vi "TSLIN_LIN_Schedule_Tab.vi"(8 "错误输入（无错误）":errorcluster, 10 "Data":T1={"Communication message"={"Sender"="", "receiver"="", "message"="", "data"=variant}, "LIN_Data"={"DLL_PATH"=path "", "Channels used"=1, "Funtiontype"=0, "Rx/TX"=enum."Rx", "Read message type"=enum."Receive&send messages", "async&sync"=enum."async", "sync_sendTimeout"=0, "LIN_SendHead"={"ALINIdxchn"=0, "ALINId"=0, "ALINDLC"=0}, "LIN_Set"={"Hardware Type"=3, "Hardware Subtype"=enum."TC1026", "AHwChannel"=0, "AAppChannel"=0, "ABaudrateKbps"=19.2, "AProtocol"=2, "AldHW"=0}, "LIN_DATA"={"Data0"=0, "Data1"=0, "Data2"=0, "Data3"=0, "Data4"=0, "Data5"=0, "Data6"=0, "Data7"=0}, "LIN_Set_Array"=[], "LDF"={"LDF Path"=path "", "LDF loading channel"=0}, "Blf_Log"={"Blf_Log_PATH"=path ""}, "LIN Scheduling Table Array"=[], "REC_Channel"=0}, "LIN Data array"=[], "error in"={"status"=FALSE, "code"=0, "source"=""}, "REC_Channel"=0, "AsynCall?"=FALSE, "DataBase_array"=refnum} {"REC_Channel" items=["CHN1", "CHN2", "CHN3", "CHN4", "CHN5", "CHN6", "CHN7", "CHN8", "CHN9", "CHN10", "CHN11", "CHN12", "CHN13", "CHN14", "CHN15", "CHN16", "CHN17", "CHN18", "CHN19", "CHN20", "CHN21", "CHN22", "CHN23", "CHN24", "CHN25", "CHN26", "CHN27", "CHN28", "CHN29", "CHN30", "CHN31", "CHN32"]; "LIN_Data"."REC_Channel" items=["CHN1", "CHN2", "CHN3", "CHN4", "CHN5", "CHN6", "CHN7", "CHN8", "CHN9", "CHN10", "CHN11", "CHN12", "CHN13", "CHN14", "CHN15", "CHN16", "CHN17", "CHN18", "CHN19", "CHN20", "CHN21", "CHN22", "CHN23", "CHN24", "CHN25", "CHN26", "CHN27", "CHN28", "CHN29", "CHN30", "CHN31", "CHN32"]; "LIN_Data"."LIN Scheduling Table Array"."LIN_Transmit"."Channel" items=["CHN1", "CHN2", "CHN3", "CHN4", "CHN5", "CHN6", "CHN7", "CHN8", "CHN9", "CHN10", "CHN11", "CHN12", "CHN13", "CHN14", "CHN15", "CHN16", "CHN17", "CHN18", "CHN19", "CHN20", "CHN21", "CHN22", "CHN23", "CHN24", "CHN25", "CHN26", "CHN27", "CHN28", "CHN29", "CHN30", "CHN31", "CHN32"]; "LIN_Data"."LIN Scheduling Table Array"."LIN_Transmit"."ID" format="%.0x"; "LIN_Data"."LIN Scheduling Table Array"."LIN_Transmit"."DLC" format="%.0x"; "LIN_Data"."LIN Scheduling Table Array"."LIN_Transmit"."Set_node_funtiontype" items=["MasterNode", "SlaveNode", "MonitorNote"]; "LIN_Data"."LDF"."LDF loading channel" items=["CHN1", "CHN2", "CHN3", "CHN4", "CHN5", "CHN6", "CHN7", "CHN8", "CHN9", "CHN10", "CHN11", "CHN12", "CHN13", "CHN14", "CHN15", "CHN16", "CHN17", "CHN18", "CHN19", "CHN20", "CHN21", "CHN22", "CHN23", "CHN24", "CHN25", "CHN26", "CHN27", "CHN28", "CHN29", "CHN30", "CHN31", "CHN32"]; "LIN_Data"."LIN_Set_Array"."Set_node_funtiontype" items=["MasterNode", "SlaveNode", "MonitorNote"]; "LIN_Data"."LIN_Set_Array"."Set"."Hardware Type" items=["BUS_UNKNOWN_TYPE", "TS_TCP_DEVICE", "XL_USB_DEVICE", "TS_USB_DEVICE", "PEAK_USB_DEVICE", "KVASER_USB_DEVICE", "ZLG_USB_DEVICE", "ICS_USB_DEVICE", "TS_TC1005_DEVICE", "CANABLE_USB_DEVICE", "TS_WIRELESS_OBD", "TS_USB_DEVICE_EX", "IXXAT_USB_DEVICE", "TS_ETH_IF_DEVICE", "TS_USB_IF_DEVICE", "BUS_DEV_TYPE_COUNT"]; "LIN_Data"."LIN_Set_Array"."Set"."AHwChannel" items=["CHN1", "CHN2", "CHN3", "CHN4", "CHN5", "CHN6", "CHN7", "CHN8", "CHN9", "CHN10", "CHN11", "CHN12", "CHN13", "CHN14", "CHN15", "CHN16", "CHN17", "CHN18", "CHN19", "CHN20", "CHN21", "CHN22", "CHN23", "CHN24", "CHN25", "CHN26", "CHN27", "CHN28", "CHN29", "CHN30", "CHN31", "CHN32"]; "LIN_Data"."LIN_Set_Array"."Set"."AAppChannel" items=["CHN1", "CHN2", "CHN3", "CHN4", "CHN5", "CHN6", "CHN7", "CHN8", "CHN9", "CHN10", "CHN11", "CHN12", "CHN13", "CHN14", "CHN15", "CHN16", "CHN17", "CHN18", "CHN19", "CHN20", "CHN21", "CHN22", "CHN23", "CHN24", "CHN25", "CHN26", "CHN27", "CHN28", "CHN29", "CHN30", "CHN31", "CHN32"]; "LIN_Data"."LIN_Set_Array"."Set"."AProtocol" items=["Lin_Protocol_13", "Lin_Protocol_20", "Lin_Protocol_21", "Lin_Protocol_J2602"]; "LIN_Data"."Funtiontype" items=["MasterNode", "SlaveNode", "MonitorNote"]; "LIN_Data"."LIN_SendHead"."ALINDLC" format="%.0x"; "LIN_Data"."LIN_SendHead"."ALINId" format="%.0x"; "LIN_Data"."LIN_SendHead"."ALINIdxchn" items=["CHN1", "CHN2", "CHN3", "CHN4", "CHN5", "CHN6", "CHN7", "CHN8", "CHN9", "CHN10", "CHN11", "CHN12", "CHN13", "CHN14", "CHN15", "CHN16", "CHN17", "CHN18", "CHN19", "CHN20", "CHN21", "CHN22", "CHN23", "CHN24", "CHN25", "CHN26", "CHN27", "CHN28", "CHN29", "CHN30", "CHN31", "CHN32"]; "LIN_Data"."LIN_Set"."Hardware Type" items=["BUS_UNKNOWN_TYPE", "TS_TCP_DEVICE", "XL_USB_DEVICE", "TS_USB_DEVICE", "PEAK_USB_DEVICE", "KVASER_USB_DEVICE", "ZLG_USB_DEVICE", "ICS_USB_DEVICE", "TS_TC1005_DEVICE", "CANABLE_USB_DEVICE", "TS_WIRELESS_OBD", "TS_USB_DEVICE_EX", "IXXAT_USB_DEVICE", "TS_ETH_IF_DEVICE", "TS_USB_IF_DEVICE", "BUS_DEV_TYPE_COUNT"]; "LIN_Data"."LIN_Set"."AHwChannel" items=["CHN1", "CHN2", "CHN3", "CHN4", "CHN5", "CHN6", "CHN7", "CHN8", "CHN9", "CHN10", "CHN11", "CHN12", "CHN13", "CHN14", "CHN15", "CHN16", "CHN17", "CHN18", "CHN19", "CHN20", "CHN21", "CHN22", "CHN23", "CHN24", "CHN25", "CHN26", "CHN27", "CHN28", "CHN29", "CHN30", "CHN31", "CHN32"]; "LIN_Data"."LIN_Set"."AAppChannel" items=["CHN1", "CHN2", "CHN3", "CHN4", "CHN5", "CHN6", "CHN7", "CHN8", "CHN9", "CHN10", "CHN11", "CHN12", "CHN13", "CHN14", "CHN15", "CHN16", "CHN17", "CHN18", "CHN19", "CHN20", "CHN21", "CHN22", "CHN23", "CHN24", "CHN25", "CHN26", "CHN27", "CHN28", "CHN29", "CHN30", "CHN31", "CHN32"]; "LIN_Data"."LIN_Set"."AProtocol" items=["Lin_Protocol_13", "Lin_Protocol_20", "Lin_Protocol_21", "Lin_Protocol_J2602"]; "LIN_Data"."Channels used" items=["1 Channel"=1, "2 Channels"=2, "3 Channels"=3, "4 Channels"=4, "5 Channels"=5]}, 11 "Sender":string="Demo") -> (0 "错误输出":errorcluster, 3 "Data out":T1={"Communication message"={"Sender"="", "receiver"="", "message"="", "data"=variant}, "LIN_Data"={"DLL_PATH"=path "", "Channels used"=1, "Funtiontype"=0, "Rx/TX"=enum."Rx", "Read message type"=enum."Receive&send messages", "async&sync"=enum."async", "sync_sendTimeout"=0, "LIN_SendHead"={"ALINIdxchn"=0, "ALINId"=0, "ALINDLC"=0}, "LIN_Set"={"Hardware Type"=3, "Hardware Subtype"=enum."TC1026", "AHwChannel"=0, "AAppChannel"=0, "ABaudrateKbps"=19.2, "AProtocol"=2, "AldHW"=0}, "LIN_DATA"={"Data0"=0, "Data1"=0, "Data2"=0, "Data3"=0, "Data4"=0, "Data5"=0, "Data6"=0, "Data7"=0}, "LIN_Set_Array"=[], "LDF"={"LDF Path"=path "", "LDF loading channel"=0}, "Blf_Log"={"Blf_Log_PATH"=path ""}, "LIN Scheduling Table Array"=[], "REC_Channel"=0}, "LIN Data array"=[], "error in"={"status"=FALSE, "code"=0, "source"=""}, "REC_Channel"=0, "AsynCall?"=FALSE, "DataBase_array"=refnum} {"REC_Channel" items=["CHN1", "CHN2", "CHN3", "CHN4", "CHN5", "CHN6", "CHN7", "CHN8", "CHN9", "CHN10", "CHN11", "CHN12", "CHN13", "CHN14", "CHN15", "CHN16", "CHN17", "CHN18", "CHN19", "CHN20", "CHN21", "CHN22", "CHN23", "CHN24", "CHN25", "CHN26", "CHN27", "CHN28", "CHN29", "CHN30", "CHN31", "CHN32"]; "LIN_Data"."REC_Channel" items=["CHN1", "CHN2", "CHN3", "CHN4", "CHN5", "CHN6", "CHN7", "CHN8", "CHN9", "CHN10", "CHN11", "CHN12", "CHN13", "CHN14", "CHN15", "CHN16", "CHN17", "CHN18", "CHN19", "CHN20", "CHN21", "CHN22", "CHN23", "CHN24", "CHN25", "CHN26", "CHN27", "CHN28", "CHN29", "CHN30", "CHN31", "CHN32"]; "LIN_Data"."LIN Scheduling Table Array"."LIN_Transmit"."Channel" items=["CHN1", "CHN2", "CHN3", "CHN4", "CHN5", "CHN6", "CHN7", "CHN8", "CHN9", "CHN10", "CHN11", "CHN12", "CHN13", "CHN14", "CHN15", "CHN16", "CHN17", "CHN18", "CHN19", "CHN20", "CHN21", "CHN22", "CHN23", "CHN24", "CHN25", "CHN26", "CHN27", "CHN28", "CHN29", "CHN30", "CHN31", "CHN32"]; "LIN_Data"."LIN Scheduling Table Array"."LIN_Transmit"."ID" format="%.0x"; "LIN_Data"."LIN Scheduling Table Array"."LIN_Transmit"."DLC" format="%.0x"; "LIN_Data"."LIN Scheduling Table Array"."LIN_Transmit"."Set_node_funtiontype" items=["MasterNode", "SlaveNode", "MonitorNote"]; "LIN_Data"."LDF"."LDF loading channel" items=["CHN1", "CHN2", "CHN3", "CHN4", "CHN5", "CHN6", "CHN7", "CHN8", "CHN9", "CHN10", "CHN11", "CHN12", "CHN13", "CHN14", "CHN15", "CHN16", "CHN17", "CHN18", "CHN19", "CHN20", "CHN21", "CHN22", "CHN23", "CHN24", "CHN25", "CHN26", "CHN27", "CHN28", "CHN29", "CHN30", "CHN31", "CHN32"]; "LIN_Data"."LIN_Set_Array"."Set_node_funtiontype" items=["MasterNode", "SlaveNode", "MonitorNote"]; "LIN_Data"."LIN_Set_Array"."Set"."Hardware Type" items=["BUS_UNKNOWN_TYPE", "TS_TCP_DEVICE", "XL_USB_DEVICE", "TS_USB_DEVICE", "PEAK_USB_DEVICE", "KVASER_USB_DEVICE", "ZLG_USB_DEVICE", "ICS_USB_DEVICE", "TS_TC1005_DEVICE", "CANABLE_USB_DEVICE", "TS_WIRELESS_OBD", "TS_USB_DEVICE_EX", "IXXAT_USB_DEVICE", "TS_ETH_IF_DEVICE", "TS_USB_IF_DEVICE", "BUS_DEV_TYPE_COUNT"]; "LIN_Data"."LIN_Set_Array"."Set"."AHwChannel" items=["CHN1", "CHN2", "CHN3", "CHN4", "CHN5", "CHN6", "CHN7", "CHN8", "CHN9", "CHN10", "CHN11", "CHN12", "CHN13", "CHN14", "CHN15", "CHN16", "CHN17", "CHN18", "CHN19", "CHN20", "CHN21", "CHN22", "CHN23", "CHN24", "CHN25", "CHN26", "CHN27", "CHN28", "CHN29", "CHN30", "CHN31", "CHN32"]; "LIN_Data"."LIN_Set_Array"."Set"."AAppChannel" items=["CHN1", "CHN2", "CHN3", "CHN4", "CHN5", "CHN6", "CHN7", "CHN8", "CHN9", "CHN10", "CHN11", "CHN12", "CHN13", "CHN14", "CHN15", "CHN16", "CHN17", "CHN18", "CHN19", "CHN20", "CHN21", "CHN22", "CHN23", "CHN24", "CHN25", "CHN26", "CHN27", "CHN28", "CHN29", "CHN30", "CHN31", "CHN32"]; "LIN_Data"."LIN_Set_Array"."Set"."AProtocol" items=["Lin_Protocol_13", "Lin_Protocol_20", "Lin_Protocol_21", "Lin_Protocol_J2602"]; "LIN_Data"."Funtiontype" items=["MasterNode", "SlaveNode", "MonitorNote"]; "LIN_Data"."LIN_SendHead"."ALINDLC" format="%.0x"; "LIN_Data"."LIN_SendHead"."ALINId" format="%.0x"; "LIN_Data"."LIN_SendHead"."ALINIdxchn" items=["CHN1", "CHN2", "CHN3", "CHN4", "CHN5", "CHN6", "CHN7", "CHN8", "CHN9", "CHN10", "CHN11", "CHN12", "CHN13", "CHN14", "CHN15", "CHN16", "CHN17", "CHN18", "CHN19", "CHN20", "CHN21", "CHN22", "CHN23", "CHN24", "CHN25", "CHN26", "CHN27", "CHN28", "CHN29", "CHN30", "CHN31", "CHN32"]; "LIN_Data"."LIN_Set"."Hardware Type" items=["BUS_UNKNOWN_TYPE", "TS_TCP_DEVICE", "XL_USB_DEVICE", "TS_USB_DEVICE", "PEAK_USB_DEVICE", "KVASER_USB_DEVICE", "ZLG_USB_DEVICE", "ICS_USB_DEVICE", "TS_TC1005_DEVICE", "CANABLE_USB_DEVICE", "TS_WIRELESS_OBD", "TS_USB_DEVICE_EX", "IXXAT_USB_DEVICE", "TS_ETH_IF_DEVICE", "TS_USB_IF_DEVICE", "BUS_DEV_TYPE_COUNT"]; "LIN_Data"."LIN_Set"."AHwChannel" items=["CHN1", "CHN2", "CHN3", "CHN4", "CHN5", "CHN6", "CHN7", "CHN8", "CHN9", "CHN10", "CHN11", "CHN12", "CHN13", "CHN14", "CHN15", "CHN16", "CHN17", "CHN18", "CHN19", "CHN20", "CHN21", "CHN22", "CHN23", "CHN24", "CHN25", "CHN26", "CHN27", "CHN28", "CHN29", "CHN30", "CHN31", "CHN32"]; "LIN_Data"."LIN_Set"."AAppChannel" items=["CHN1", "CHN2", "CHN3", "CHN4", "CHN5", "CHN6", "CHN7", "CHN8", "CHN9", "CHN10", "CHN11", "CHN12", "CHN13", "CHN14", "CHN15", "CHN16", "CHN17", "CHN18", "CHN19", "CHN20", "CHN21", "CHN22", "CHN23", "CHN24", "CHN25", "CHN26", "CHN27", "CHN28", "CHN29", "CHN30", "CHN31", "CHN32"]; "LIN_Data"."LIN_Set"."AProtocol" items=["Lin_Protocol_13", "Lin_Protocol_20", "Lin_Protocol_21", "Lin_Protocol_J2602"]; "LIN_Data"."Channels used" items=["1 Channel"=1, "2 Channels"=2, "3 Channels"=3, "4 Channels"=4, "5 Channels"=5]})   [LabVIEW 2014]
uses:
  Typedef/TSLIN_Transmit.ctl
  Typedef/TSLIN_LIN Schedule_Table.ctl
  Typedef/TSLIN_SendHead.ctl
  Utilities/Typedef/Hardware_Subtype.ctl
  Typedef/TSLIN_SetData.ctl
  Typedef/TSLIN_Config.ctl
  Typedef/TLibLIN.ctl
  Typedef/TSLIN_Data.ctl
  <vilib>/Utility/miscctls.llb/LVPointTypeDef.ctl
  Typedef/TSLIN_LIN_Set.ctl
  All_Control/Typedef/Hardware Type.ctl
  All_Control/Typedef/Blf_Log.ctl
  DataBase/Typedef/DataBase_array_index.ctl
  DataBase/Typedef/CAN/TCANSignal.ctl
  DataBase/Typedef/LIN/TLINSignal.ctl
  DataBase/Typedef/FlexRay/TFlexRaySignal.ctl
  DataBase/Typedef/TDBSignalProperties.ctl
  DataBase/Typedef/TDBFrameProperties.ctl
  DataBase/Typedef/TDBECUProperties.ctl
  DataBase/Typedef/TDBProperties.ctl
  DataBase/Typedef/DataBase_array.ctl
panel:
  in  "Signals":string[][](array[string])
  in  "Messages":string(combo)
  out "result 3":bool
  in  "Clear CH":bool
  out "result 2":bool
  out "result":bool
  in  "LIN_Data_display":i32(listbox)
  in  "LIN scheduling table":T9 {"LIN_Transmit"."FDatas"."value 7" format="%.0x"; "LIN_Transmit"."FDatas"."value 6" format="%.0x"; "LIN_Transmit"."FDatas"."value 5" format="%.0x"; "LIN_Transmit"."FDatas"."value 4" format="%.0x"; "LIN_Transmit"."FDatas"."value 3" format="%.0x"; "LIN_Transmit"."FDatas"."value 2" format="%.0x"; "LIN_Transmit"."FDatas"."value 1" format="%.0x"; "LIN_Transmit"."FDatas"."value0" format="%.0x"; "LIN_Transmit"."Channel" items=["CHN1", "CHN2", "CHN3", "CHN4", "CHN5", "CHN6", "CHN7", "CHN8", "CHN9", "CHN10", "CHN11", "CHN12", "CHN13", "CHN14", "CHN15", "CHN16", "CHN17", "CHN18", "CHN19", "CHN20", "CHN21", "CHN22", "CHN23", "CHN24", "CHN25", "CHN26", "CHN27", "CHN28", "CHN29", "CHN30", "CHN31", "CHN32"]; "LIN_Transmit"."ID" format="%.0x"; "LIN_Transmit"."Set_node_funtiontype" items=["MasterNode", "SlaveNode", "MonitorNote"]}
  in  "Clear all":bool
  in  "Add":bool
  in  "Confirm":bool
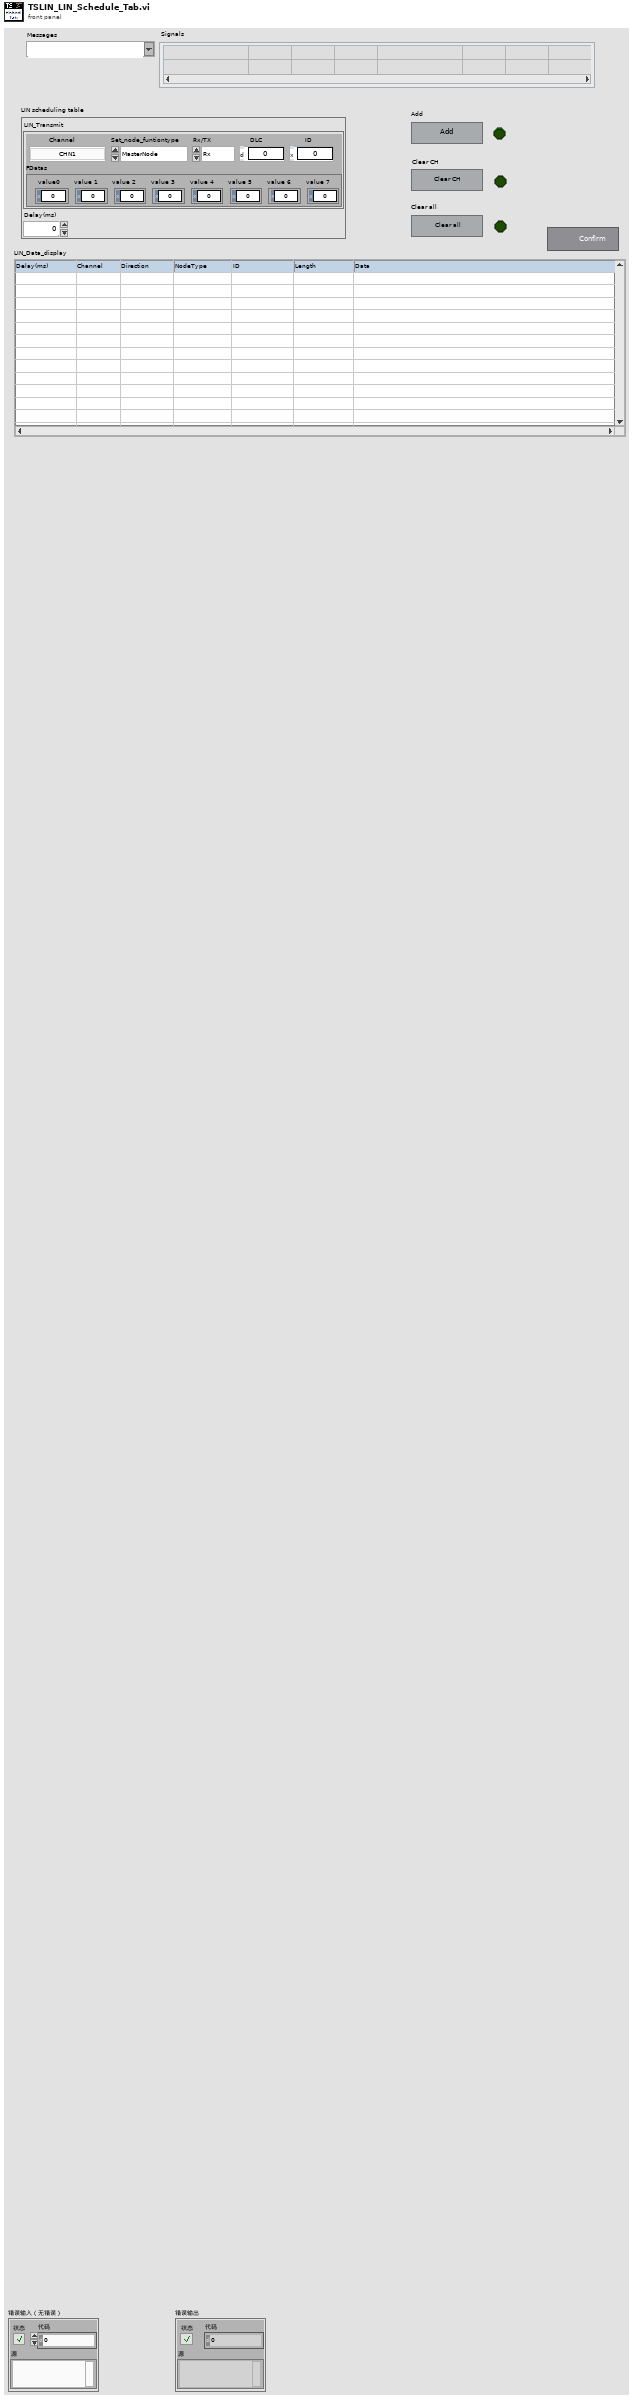
[diagram p1: front panel]
types:
  T1 = typedef "TSLIN_Data.ctl" = cluster{"Communication message":cluster{"Sender":string, "receiver":string, "message":string, "data":variant}, "LIN_Data":T2, "LIN Data array":T11[], "error in":errorcluster, "REC_Channel":i32, "AsynCall?":bool, "DataBase_array":T12}
  T2 = typedef "TSLIN_Config.ctl" = cluster{"DLL_PATH":path, "Channels used":u16, "Funtiontype":i32, "Rx/TX":enum16{"Rx", "Tx"}, "Read message type":enum16{"Only read received messages", "Receive&send messages"}, "async&sync":enum16{"async", "sync"}, "sync_sendTimeout":u16, "LIN_SendHead":T3, "LIN_Set":T4, "LIN_DATA":cluster{"Data0":u8, "Data1":u8, "Data2":u8, "Data3":u8, "Data4":u8, "Data5":u8, "Data6":u8, "Data7":u8}, "LIN_Set_Array":T7[], "LDF":cluster{"LDF Path":path, "LDF loading channel":i32}, "Blf_Log":T8, "LIN Scheduling Table Array":T9[], "REC_Channel":i32}
  T3 = typedef "TSLIN_SendHead.ctl" = cluster{"ALINIdxchn":u8, "ALINId":u32, "ALINDLC":u32}
  T4 = typedef "TSLIN_SetData.ctl" = cluster{"Hardware Type":T5, "Hardware Subtype":T6, "AHwChannel":i32, "AAppChannel":i32, "ABaudrateKbps":sgl, "AProtocol":i32, "AldHW":i32}
  T5 = typedef "Hardware Type.ctl" = i32
  T6 = typedef "Hardware_Subtype.ctl" = enum16{"TS_UNKNOWN_DEVICE", "TSCAN_PRO", "TSCAN_Lite1", "TC1001", "TL1001", "TC1011", "TM5011", "TC1002", "TC1014", "TSCANFD2517", "TC1026", "TC1016", "TC1012", "TC1013", "TLog1002", "TC1034", "TC1018", "GW2116", "TC2115", "MP1013", "TC1113", "TC1114", "TP1013", "TC1017", "TP1018", "TF10XX", "TL1004_FD_4_LIN_2", "TE1051", "TP1051", "TP1034", "TTS9015", "TP1026", "TTS1026", "TTS1034", "TTS1018", "TL1011", "TTS1015_LiAuto", "TTS1013_LiAuto", "TTS1016Pro", "TC1054Pro", "TC1054", "TLog1038", "TO1013", "TC1034Pro", "TC1018Pro", "TC1038Pro", "TS_DEV_END"}
  T7 = typedef "TSLIN_LIN_Set.ctl" = cluster{"Set":T4, "Set_node_funtiontype":i32}
  T8 = typedef "Blf_Log.ctl" = cluster{"Blf_Log_PATH":path}
  T9 = typedef "TSLIN_LIN Schedule_Table.ctl" = cluster{"LIN_Transmit":T10, "Delay(ms)":i32}
  T10 = typedef "TSLIN_Transmit.ctl" = cluster{"Channel":i32, "Rx/TX":enum16{"Rx", "Tx"}, "Set_node_funtiontype":i32, "DLC":u32, "ID":u32, "FDatas":cluster{"value0":u8, "value 1":u8, "value 2":u8, "value 3":u8, "value 4":u8, "value 5":u8, "value 6":u8, "value 7":u8}}
  T11 = typedef "TLibLIN.ctl" = cluster{"Ch":u8, "Code":u8, "Properties":u8, "FDLC":u8, "ID":u8, "Checksum":u8, "FStaus":u8, "FTimeUS":u64, "FDatas":cluster{"value0":u8, "value 1":u8, "value 2":u8, "value 3":u8, "value 4":u8, "value 5":u8, "value 6":u8, "value 7":u8}}
  T12 = typedef "DataBase_array_index.ctl" = refnum<vi>
  T13 = cluster{"Sender":string, "receiver":string, "message":string, "data":variant}
  T14 = typedef "LVPointTypeDef.ctl" = cluster{"Horizontal":i16, "Vertical":i16}
  T15 = typedef "TDBFrameProperties.ctl" = cluster{"FDBIndex":i32, "FECUIndex":i32, "FFrameIndex":i32, "FIsTx":u8, "FReserved1":u8, "FCycleTimeMs":u16, "TSignalType":i32, "FCANIsDataFrame":u8, "FCANIsStdFrame":u8, "FCANIsEdl":u8, "FCANIsBrs":u8, "FCANIdentifier":i32, "FCANDLC":i32, "FCANDataBytes":i32, "FLINIdentifier":i32, "FLINDLC":i32, "FFRChannelMask":u8, "FFRBaseCycle":u8, "FFRCycleRepetition":u8, "FFRIsStartupFrame":u8, "FFRSlotId":u16, "FFRDLC":u16, "FFRCycleMask":u64, "FSignalCount":i32, "FName":cluster{"数值":u64, "数值 2":u64, "数值 3":u64, "数值 4":u64, "数值 5":u64, "数值 6":u64, "数值 7":u64, "数值 8":u64, "数值 9":u64, "数值 10":u64, "数值 11":u64, "数值 12":u64, "数值 13":u64, "数值 14":u64, "数值 15":u64, "数值 16":u64, "数值 17":u64, "数值 18":u64, "数值 19":u64, "数值 20":u64, "数值 21":u64, "数值 22":u64, "数值 23":u64, "数值 24":u64, "数值 25":u64, "数值 26":u64, "数值 27":u64, "数值 28":u64, "数值 29":u64, "数值 30":u64, "数值 31":u64, "数值 32":u64, "数值 33":u64, "数值 34":u64, "数值 35":u64, "数值 36":u64, "数值 37":u64, "数值 38":u64, "数值 39":u64, "数值 40":u64, "数值 41":u64, "数值 42":u64, "数值 43":u64, "数值 44":u64, "数值 45":u64, "数值 46":u64, "数值 47":u64, "数值 48":u64, "数值 49":u64, "数值 50":u64, "数值 51":u64, "数值 52":u64, "数值 53":u64, "数值 54":u64, "数值 55":u64, "数值 56":u64, "数值 57":u64, "数值 58":u64, "数值 59":u64, "数值 60":u64, "数值 61":u64, "数值 62":u64, "数值 63":u64, "数值 64":u64}, "FComment":cluster{"数值":u64, "数值 2":u64, "数值 3":u64, "数值 4":u64, "数值 5":u64, "数值 6":u64, "数值 7":u64, "数值 8":u64, "数值 9":u64, "数值 10":u64, "数值 11":u64, "数值 12":u64, "数值 13":u64, "数值 14":u64, "数值 15":u64, "数值 16":u64, "数值 17":u64, "数值 18":u64, "数值 19":u64, "数值 20":u64, "数值 21":u64, "数值 22":u64, "数值 23":u64, "数值 24":u64, "数值 25":u64, "数值 26":u64, "数值 27":u64, "数值 28":u64, "数值 29":u64, "数值 30":u64, "数值 31":u64, "数值 32":u64, "数值 33":u64, "数值 34":u64, "数值 35":u64, "数值 36":u64, "数值 37":u64, "数值 38":u64, "数值 39":u64, "数值 40":u64, "数值 41":u64, "数值 42":u64, "数值 43":u64, "数值 44":u64, "数值 45":u64, "数值 46":u64, "数值 47":u64, "数值 48":u64, "数值 49":u64, "数值 50":u64, "数值 51":u64, "数值 52":u64, "数值 53":u64, "数值 54":u64, "数值 55":u64, "数值 56":u64, "数值 57":u64, "数值 58":u64, "数值 59":u64, "数值 60":u64, "数值 61":u64, "数值 62":u64, "数值 63":u64, "数值 64":u64}}
  T16 = typedef "TDBSignalProperties.ctl" = cluster{"FDBIndex":i32, "FECUIndex":i32, "FFrameIndex":i32, "FSignalIndex":i32, "FIsTx":u8, "FReserved1":u8, "FReserved2":u8, "FReserved3":u8, "TSignalType":i32, "TCANSignal":T17, "TLINSignal":T18, "TFlexRaySignal":T19, "FParentFrameId":i32, "FInitValue":dbl, "FName":cluster{"数值":u64, "数值 2":u64, "数值 3":u64, "数值 4":u64, "数值 5":u64, "数值 6":u64, "数值 7":u64, "数值 8":u64, "数值 9":u64, "数值 10":u64, "数值 11":u64, "数值 12":u64, "数值 13":u64, "数值 14":u64, "数值 15":u64, "数值 16":u64, "数值 17":u64, "数值 18":u64, "数值 19":u64, "数值 20":u64, "数值 21":u64, "数值 22":u64, "数值 23":u64, "数值 24":u64, "数值 25":u64, "数值 26":u64, "数值 27":u64, "数值 28":u64, "数值 29":u64, "数值 30":u64, "数值 31":u64, "数值 32":u64, "数值 33":u64, "数值 34":u64, "数值 35":u64, "数值 36":u64, "数值 37":u64, "数值 38":u64, "数值 39":u64, "数值 40":u64, "数值 41":u64, "数值 42":u64, "数值 43":u64, "数值 44":u64, "数值 45":u64, "数值 46":u64, "数值 47":u64, "数值 48":u64, "数值 49":u64, "数值 50":u64, "数值 51":u64, "数值 52":u64, "数值 53":u64, "数值 54":u64, "数值 55":u64, "数值 56":u64, "数值 57":u64, "数值 58":u64, "数值 59":u64, "数值 60":u64, "数值 61":u64, "数值 62":u64, "数值 63":u64, "数值 64":u64}, "FComment":cluster{"数值":u64, "数值 2":u64, "数值 3":u64, "数值 4":u64, "数值 5":u64, "数值 6":u64, "数值 7":u64, "数值 8":u64, "数值 9":u64, "数值 10":u64, "数值 11":u64, "数值 12":u64, "数值 13":u64, "数值 14":u64, "数值 15":u64, "数值 16":u64, "数值 17":u64, "数值 18":u64, "数值 19":u64, "数值 20":u64, "数值 21":u64, "数值 22":u64, "数值 23":u64, "数值 24":u64, "数值 25":u64, "数值 26":u64, "数值 27":u64, "数值 28":u64, "数值 29":u64, "数值 30":u64, "数值 31":u64, "数值 32":u64, "数值 33":u64, "数值 34":u64, "数值 35":u64, "数值 36":u64, "数值 37":u64, "数值 38":u64, "数值 39":u64, "数值 40":u64, "数值 41":u64, "数值 42":u64, "数值 43":u64, "数值 44":u64, "数值 45":u64, "数值 46":u64, "数值 47":u64, "数值 48":u64, "数值 49":u64, "数值 50":u64, "数值 51":u64, "数值 52":u64, "数值 53":u64, "数值 54":u64, "数值 55":u64, "数值 56":u64, "数值 57":u64, "数值 58":u64, "数值 59":u64, "数值 60":u64, "数值 61":u64, "数值 62":u64, "数值 63":u64, "数值 64":u64}}
  T17 = typedef "TCANSignal.ctl" = cluster{"FCANSgnType":u8, "FIsIntel":u8, "FStartBit":i32, "FLength":i32, "FFactor":dbl, "FOffset":dbl}
  T18 = typedef "TLINSignal.ctl" = cluster{"FLINSgnType":u8, "FIsIntel":u8, "FStartBit":i32, "FLength":i32, "FFactor":dbl, "FOffset":dbl}
  T19 = typedef "TFlexRaySignal.ctl" = cluster{"FFRSgnType":u8, "FCompuMethod":u8, "FReserved":u8, "FIsIntel":u8, "FStartBit":i32, "FUpdateBit":i32, "FLength":i32, "FFactor":dbl, "FOffset":dbl, "FActualStartBit":i32, "FActualUpdateBit":i32}
  T20 = cluster{"Frame_Properties":T15, "signal_array":T16[]}
  T21 = cluster{"Data0":u8, "Data1":u8, "Data2":u8, "Data3":u8, "Data4":u8, "Data5":u8, "Data6":u8, "Data7":u8}
  T22 = cluster{"[0]":u8, "[1]":u8, "[2]":u8, "[3]":u8, "[4]":u8, "[5]":u8, "[6]":u8, "[7]":u8}
  T23 = cluster{"value0":u8, "value 1":u8, "value 2":u8, "value 3":u8, "value 4":u8, "value 5":u8, "value 6":u8, "value 7":u8}
  T24 = enum32{"invalid app kind", "Development System", "Run Time System", "Student Edition", "Embedded LabVIEW", "Evaluation", "Custom"}
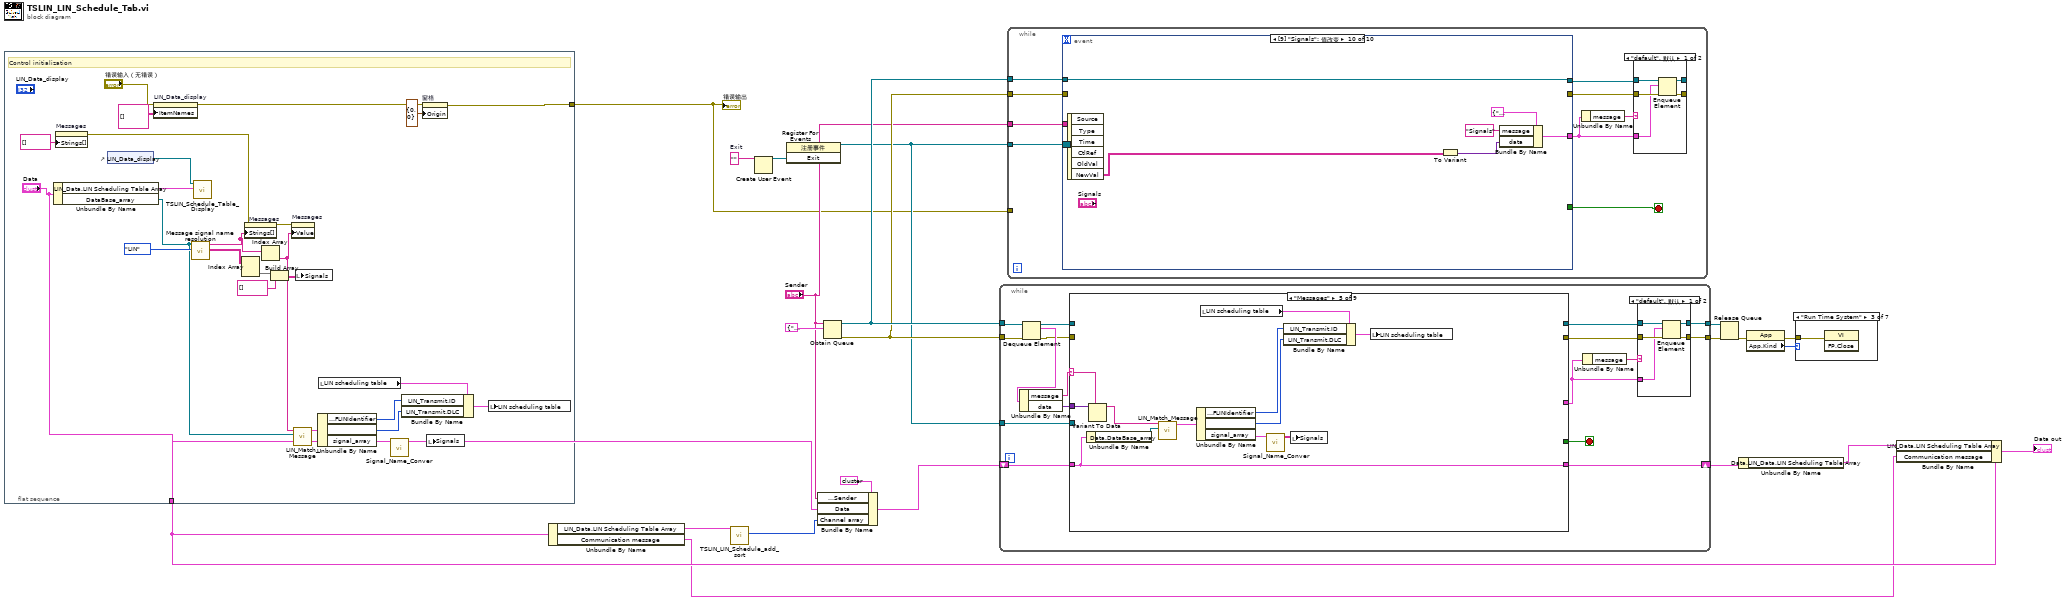
[diagram p0: block diagram]
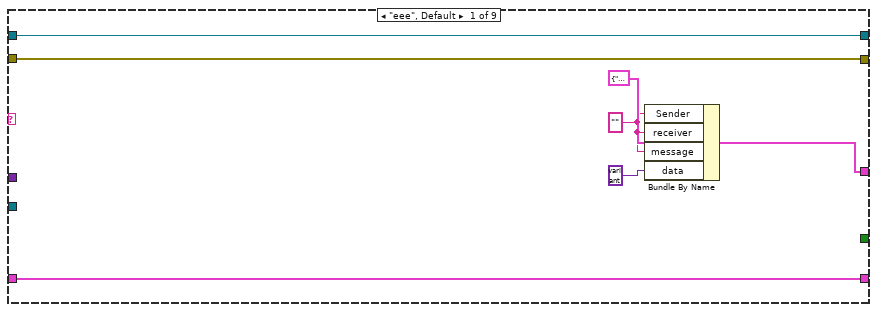
[diagram p9: hidden frame]
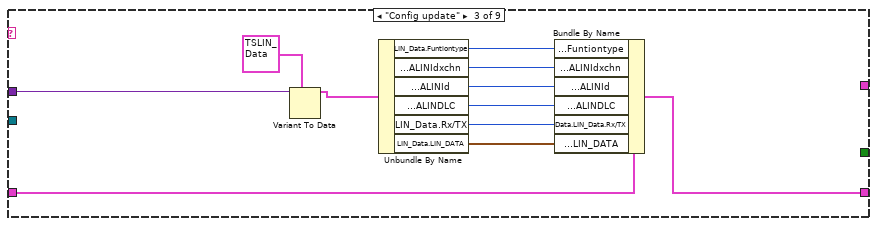
[diagram p11: hidden frame]
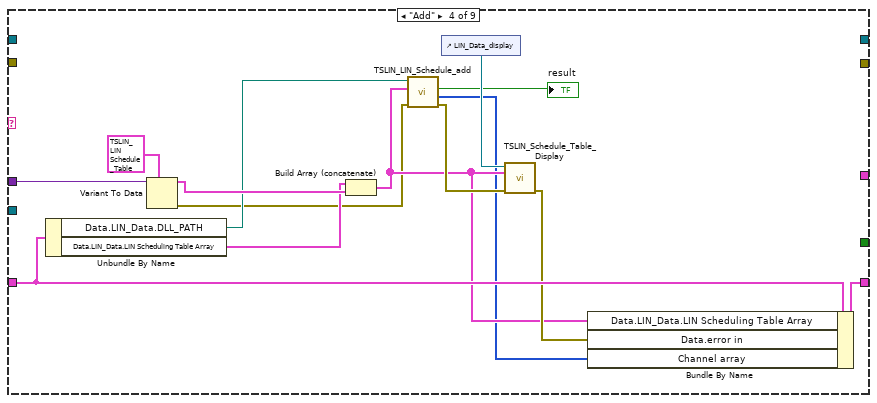
[diagram p12: hidden frame]
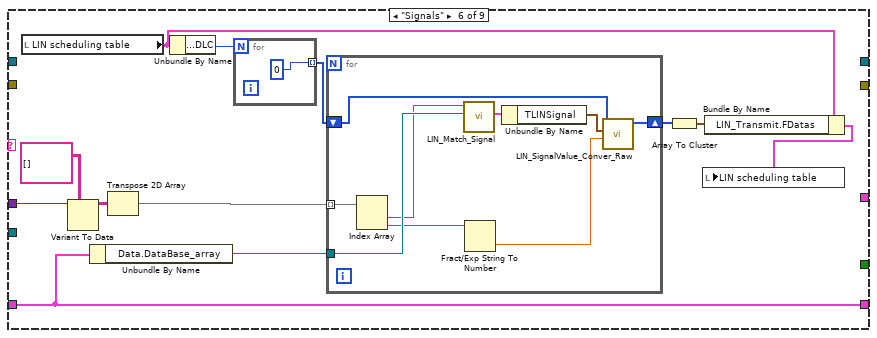
[diagram p13: hidden frame]
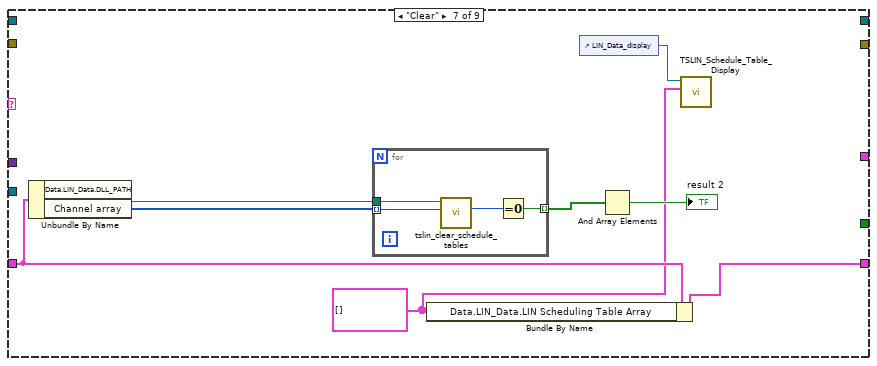
[diagram p14: hidden frame]
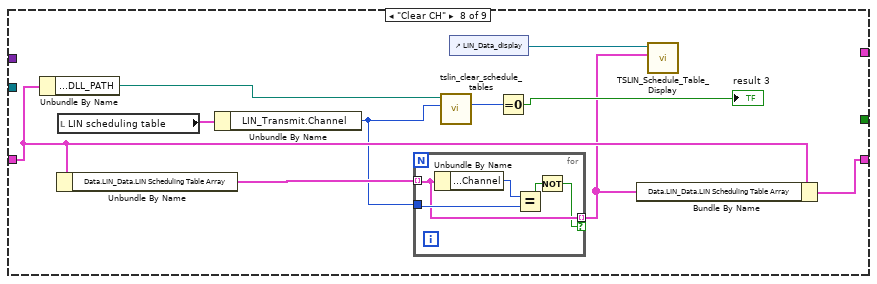
[diagram p15: hidden frame]
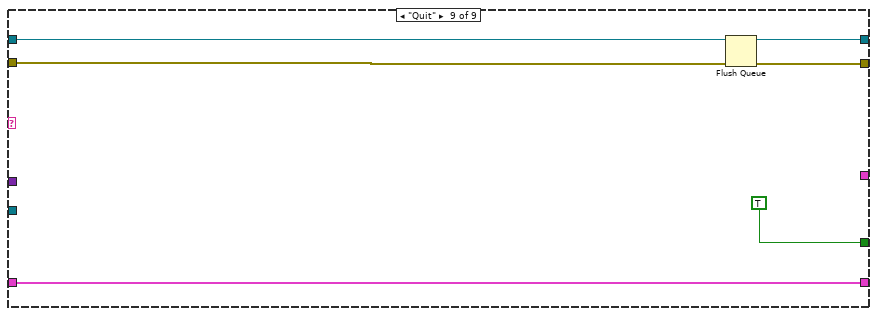
[diagram p16: hidden frame]
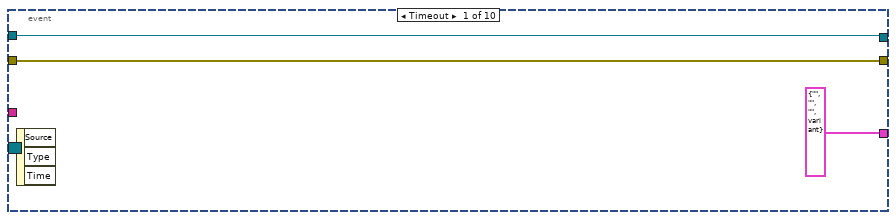
[diagram p18: hidden frame]
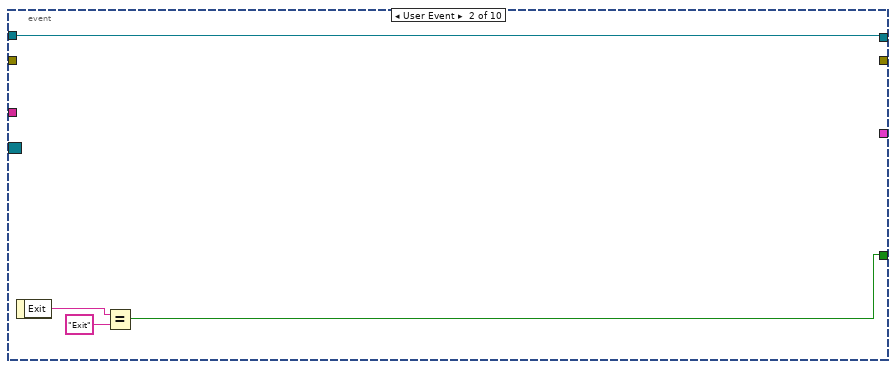
[diagram p19: hidden frame]
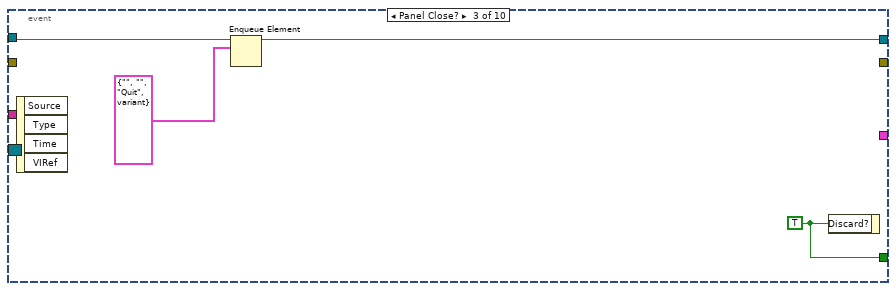
[diagram p20: hidden frame]
diagram:
  w11 = ""  # Exit
  n1 = flat-sequence {
    tunnel: [w48] -> w9
    tunnel: ["Data"] -> w4
    frame #0 {
      # "Control initialization"
      n2 = Unbundle By Name("Data") -> ("LIN_Data.LIN Scheduling Table Array"=w44:T9[], "DataBase_array"=w23:T12)
      n3 = property on="Messages" class="CmbBox"("Strings[]"=string[] [] ("字符串[]")) -> (error out=w34:errorcluster)  [unwired: 2 in, 1 out]
      n4 = control-ref of="LIN_Data_display"() -> (w45:refnum<vi>)
      n5 = property on="LIN_Data_display" class="MCListbox (严格)"(error in="错误输入（无错误）", "ItemNames"=string[][] [] ("项名")) -> (error out=w46:errorcluster)  [unwired: 1 in, 1 out]
      n6 = call "Message signal name resolution.vi"("BusType"=enum16{"LIN", "FlexRay"}."LIN", "DataBase_array"=w23) -> ("Signals Name array"=w37:string[][], "Frame Name array"=w41:string[])  [unwired: 7 in, 1 out]
      n7 = call "TSLIN_Schedule_Table_Display.vi"("LIN Scheduling Table Array"=w44, "LIN_Data Ref"=w45) -> ()  [unwired: 9 in, 1 out]
      n8 = Index Array(array=w37) -> (element=w39:string[])  [unwired: 2 in]
      n9 = property on="Messages" class="CmbBox"(error in=w34, "Strings[]"=w41) -> (error out=w40:errorcluster)  [unwired: 1 in, 1 out]
      n10 = Index Array(array=w41) -> (element=w25:string)  [unwired: 1 in]
      n11 = Build Array(w39, string[] [] ("元素")) -> (w36:string[][])
      n12 = property on="Messages" class="CmbBox"(error in=w40, "Value"=w25) -> ()  [unwired: 1 in, 2 out]
      n13 = call "LIN_Match_Message.vi"("DataBase_array"=w23, "Message"=w25) -> ("Frame"=w27:T20)  [unwired: 9 in]
      n14 = local write "Signals"(w36) -> ()
      n15 = Unbundle By Name(w27) -> ("Frame_Properties.FLINIdentifier"=w31:i32, "Frame_Properties.FLINDLC"=w32:i32, "signal_array"=w28:T16[])
      n16 = local read "LIN scheduling table"() -> (w29:T9)
      n17 = call "Signal_Name_Conver.vi"("signal_array"=w28) -> ("Signals"=w33:string[][])  [unwired: 10 in]
      n18 = Bundle By Name(cluster=w29, "LIN_Transmit.ID"=w31, "LIN_Transmit.DLC"=w32) -> (w30:T9)
      n19 = property on="窗格" class="Pane"(error in=w46, "Origin"=T14 {"Horizontal"=0, "Vertical"=0} ("原点")) -> (error out=w48:errorcluster)  [unwired: 1 in, 1 out]
      n20 = local write "Signals"(w33) -> ()
      n21 = local write "LIN scheduling table"(w30) -> ()
    }
  }
  n22 = Unbundle By Name(w4) -> ("LIN_Data.LIN Scheduling Table Array"=w3:T9[], "Communication message"=w1:T13)
  n23 = call "TSLIN_LIN_Schedule_add_sort.vi"("LIN Scheduling Table Array"=w3) -> ("CH_array"=w2:i32[])  [unwired: 9 in, 1 out]
  n24 = Create User Event(user event datatype=w11) -> (user event=w12:refnum<user-event>)  [unwired: 1 in, 1 out]
  n25 = register-events(w12) -> (reference out=w10:refnum<event-registration>)  [unwired: 2 in, 1 out]
  n26 = Bundle By Name(cluster=cluster{"Data":T1, "Channel array":i32[]} {"Data"={"Communication message"={"Sender"="", "receiver"="", "message"="", "data"=variant}, "LIN_Data"={"DLL_PATH"=path "", "Channels used"=0, "Funtiontype"=0, "Rx/TX"=enum."Rx", "Read message type"=enum."Only read received messages", "async&sync"=enum."async", "sync_sendTimeout"=0, "LIN_SendHead"={"ALINIdxchn"=0, "ALINId"=0, "ALINDLC"=0}, "LIN_Set"={"Hardware Type"=0, "Hardware Subtype"=enum."TS_UNKNOWN_DEVICE", "AHwChannel"=0, "AAppChannel"=0, "ABaudrateKbps"=0.0, "AProtocol"=0, "AldHW"=0}, "LIN_DATA"={"Data0"=0, "Data1"=0, "Data2"=0, "Data3"=0, "Data4"=0, "Data5"=0, "Data6"=0, "Data7"=0}, "LIN_Set_Array"=[], "LDF"={"LDF Path"=path "", "LDF loading channel"=0}, "Blf_Log"={"Blf_Log_PATH"=path ""}, "LIN Scheduling Table Array"=[], "REC_Channel"=0}, "LIN Data array"=[], "error in"={"status"=FALSE, "code"=0, "source"=""}, "REC_Channel"=0, "AsynCall?"=FALSE, "DataBase_array"=refnum}, "Channel array"=[]}, "Data.Communication message.Sender"="Sender", "Data"=w4, "Channel array"=w2) -> (w14:cluster{"Data":T1, "Channel array":i32[]})
  n27 = Obtain Queue(name (unnamed)="Sender", element data type=T13 {"Sender"="", "receiver"="", "message"="", "data"=variant} ("Communication message")) -> (queue out=w22:refnum<queue>, error out=w15:errorcluster)  [unwired: 3 in, 1 out]
  n28 = while {
    tunnel: w22 -> [w65]
    tunnel: w15 -> [w64]
    tunnel: [w56] -> w21
    tunnel: [w55] -> w20
    shift-right: [w50] -> w7
    shift-left: w14 -> [w51]
    tunnel: w10 -> [w49]
    stop <- w54 stop-if-true
    n29 = Dequeue Element(queue=w65, error in (no error)=w64) -> (queue out=w61:refnum<queue>, element=w63:T13, error out=w60:errorcluster)  [unwired: 1 in, 1 out]
    n30 = Unbundle By Name(w63) -> ("message"=w62:string, "data"=w57:variant)
    n31 = case shown="\"Messages\"" w62 {
      selector: w62 -> [_ _ _ _ w118 _ _ _ _]
      tunnel: [w79 w82 _ _ _ _ _ _ w173] -> w59
      tunnel: w61 -> [w79 w82 _ _ _ _ _ _ w172]
      tunnel: w60 -> [w78 w81 _ _ _ _ _ _ w170]
      tunnel: [w78 w81 _ _ _ _ _ _ w171] -> w58
      tunnel: w57 -> [_ _ w92 w106 w119 w131 _ _ _]
      tunnel: [_ _ _ _ _ _ _ _ TRUE] -> w54
      tunnel: [w76 _ _ _ _ _ _ _ _] -> w53
      tunnel: [w73 w80 w89 w107 w116 w128 w147 w156 w169] -> w50
      tunnel: w51 -> [w73 w80 w93 w104 w116 w128 w149 w158 w169]
      tunnel: w49 -> [_ _ _ _ _ _ _ _ _]
      frame "eee", Default {
        w74 = ""
        n32 = Bundle By Name(cluster=T13 {"Sender"="", "receiver"="", "message"="", "data"=variant} ("Communication message"), "Sender"=w74, "receiver"=w74, "message"=w74, "data"=variant) -> (w76:T13)
      }
      frame "Init" {
      }
      frame "Config update" {
        n33 = Variant To Data(type=T1 {"Communication message"={"Sender"="", "receiver"="", "message"="", "data"=variant}, "LIN_Data"={"DLL_PATH"=path "", "Channels used"=0, "Funtiontype"=0, "Rx/TX"=enum."Rx", "Read message type"=enum."Only read received messages", "async&sync"=enum."async", "sync_sendTimeout"=0, "LIN_SendHead"={"ALINIdxchn"=0, "ALINId"=0, "ALINDLC"=0}, "LIN_Set"={"Hardware Type"=0, "Hardware Subtype"=enum."TS_UNKNOWN_DEVICE", "AHwChannel"=0, "AAppChannel"=0, "ABaudrateKbps"=0.0, "AProtocol"=0, "AldHW"=0}, "LIN_DATA"={"Data0"=0, "Data1"=0, "Data2"=0, "Data3"=0, "Data4"=0, "Data5"=0, "Data6"=0, "Data7"=0}, "LIN_Set_Array"=[], "LDF"={"LDF Path"=path "", "LDF loading channel"=0}, "Blf_Log"={"Blf_Log_PATH"=path ""}, "LIN Scheduling Table Array"=[], "REC_Channel"=0}, "LIN Data array"=[], "error in"={"status"=FALSE, "code"=0, "source"=""}, "REC_Channel"=0, "AsynCall?"=FALSE, "DataBase_array"=refnum} ("Data"), Variant=w92) -> (data=w90:T1)  [unwired: 1 in, 1 out]
        n34 = Unbundle By Name(w90) -> ("LIN_Data.Funtiontype"=w83:i32, "LIN_Data.LIN_SendHead.ALINIdxchn"=w88:u8, "LIN_Data.LIN_SendHead.ALINId"=w87:u32, "LIN_Data.LIN_SendHead.ALINDLC"=w86:u32, "LIN_Data.Rx/TX"=w85:enum16{"Rx", "Tx"}, "LIN_Data.LIN_DATA"=w84:T21)
        n35 = Bundle By Name(cluster=w93, "Data.LIN_Data.Funtiontype"=w83, "Data.LIN_Data.LIN_SendHead.ALINIdxchn"=w88, "Data.LIN_Data.LIN_SendHead.ALINId"=w87, "Data.LIN_Data.LIN_SendHead.ALINDLC"=w86, "Data.LIN_Data.Rx/TX"=w85, "Data.LIN_Data.LIN_DATA"=w84) -> (w89:cluster{"Data":T1, "Channel array":i32[]})
      }
      frame "Add" {
        n36 = Unbundle By Name(w104) -> ("Data.LIN_Data.DLL_PATH"=w100:path, "Data.LIN_Data.LIN Scheduling Table Array"=w98:T9[])
        n37 = Variant To Data(type=T9 {"LIN_Transmit"={"Channel"=0, "Rx/TX"=enum."Rx", "Set_node_funtiontype"=0, "DLC"=0, "ID"=0, "FDatas"={"value0"=0, "value 1"=0, "value 2"=0, "value 3"=0, "value 4"=0, "value 5"=0, "value 6"=0, "value 7"=0}}, "Delay(ms)"=0} ("LIN scheduling table"), Variant=w106) -> (data=w101:T9, error out=w94:errorcluster)  [unwired: 1 in]
        n38 = Build Array (concatenate)(w98, w101) -> (w96:T9[])
        n39 = call "TSLIN_LIN_Schedule_add.vi"("错误输入"=w94, "LIN Scheduling Table Array"=w96, "路径输入"=w100) -> ("错误输出"=w97:errorcluster, "Channel array"=w95:i32[], "Successful?"=→"result":bool)  [unwired: 5 in, 1 out]
        n40 = control-ref of="LIN_Data_display"() -> (w103:refnum<vi>)
        n41 = call "TSLIN_Schedule_Table_Display.vi"("错误输入（无错误）"=w97, "LIN Scheduling Table Array"=w96, "LIN_Data Ref"=w103) -> ("错误输出"=w102:errorcluster)  [unwired: 8 in]
        n42 = Bundle By Name(cluster=w104, "Data.LIN_Data.LIN Scheduling Table Array"=w96, "Data.error in"=w102, "Channel array"=w95) -> (w107:cluster{"Data":T1, "Channel array":i32[]})
      }
      frame "Messages" {
        n43 = Unbundle By Name(w116) -> ("Data.DataBase_array"=w115:T12)
        n44 = Variant To Data(type=w118, Variant=w119) -> (data=w117:string)  [unwired: 1 in, 1 out]
        n45 = call "LIN_Match_Message.vi"("DataBase_array"=w115, "Message"=w117) -> ("Frame"=w114:T20)  [unwired: 9 in]
        n46 = Unbundle By Name(w114) -> ("Frame_Properties.FLINIdentifier"=w111:i32, "Frame_Properties.FLINDLC"=w110:i32, "signal_array"=w109:T16[])
        n47 = local read "LIN scheduling table"() -> (w113:T9)
        n48 = call "Signal_Name_Conver.vi"("signal_array"=w109) -> ("Signals"=w108:string[][])  [unwired: 10 in]
        n49 = Bundle By Name(cluster=w113, "LIN_Transmit.ID"=w111, "LIN_Transmit.DLC"=w110) -> (w112:T9)
        n50 = local write "Signals"(w108) -> ()
        n51 = local write "LIN scheduling table"(w112) -> ()
      }
      frame "Signals" {
        n52 = local read "LIN scheduling table"() -> (w123:T9)
        n53 = Variant To Data(type=string[][] [] ("新值"), Variant=w131) -> (data=w129:string[][])  [unwired: 1 in, 1 out]
        n54 = Unbundle By Name(w128) -> ("Data.DataBase_array"=w127:T12)
        n55 = Transpose 2D Array(2D array=w129) -> (transposed array=w126:string[][])
        n56 = Unbundle By Name(w123) -> ("LIN_Transmit.DLC"=w125:u32)
        n57 = for {
          N: w125 -> [_]
          tunnel: [u8 0] -> w124 mode=indexing
        }
        n58 = for {
          tunnel: w126 -> [w141] mode=indexing
          tunnel: w127 -> [w140]
          shift-right: [w138] -> w121
          shift-left: w124 -> [w137]
          n59 = Index Array(array=w141) -> (element #1=w136:string, element #2=w133:string)  [unwired: 2 in]
          n60 = call "LIN_Match_Signal.vi"("DataBase_array"=w140, "Signal"=w136) -> ("TDBSignalProperties"=w139:T16)  [unwired: 9 in]
          n61 = Fract/Exp String To Number(string=w133) -> (number=w135:dbl)  [unwired: 3 in, 1 out]
          n62 = Unbundle By Name(w139) -> ("TLINSignal"=w134:T18)
          n63 = call "LIN_SignalValue_Conver_Raw.vi"("Signal_Value"=w135, "TLINSignal"=w134, "data in"=w137) -> ("data"=w138:u8[])  [unwired: 8 in]
        }
        n64 = Array To Cluster(array=w121) -> (cluster=w120:T22)
        n65 = Bundle By Name(cluster=w123, "LIN_Transmit.FDatas"=w120) -> (w122:T9)
        n66 = local write "LIN scheduling table"(w122) -> ()
      }
      frame "Clear" {
        w142 = T9[] [] ("LIN Scheduling Table Array")
        n67 = Unbundle By Name(w149) -> ("Data.LIN_Data.DLL_PATH"=w148:path, "Channel array"=w145:i32[])
        n68 = for {
          tunnel: w148 -> [w153]
          tunnel: w145 -> [w152] mode=indexing
          tunnel: [w150] -> w146 mode=indexing
          n69 = call "tslin_clear_schedule_tables.vi"("ALdxChn"=w152, "路径输入"=w153) -> ("return"=w151:i32)  [unwired: 7 in, 2 out]
          n70 = Equal To 0?(x=w151) -> (x = 0?=w150:bool)
        }
        n71 = Bundle By Name(cluster=w149, "Data.LIN_Data.LIN Scheduling Table Array"=w142) -> (w147:cluster{"Data":T1, "Channel array":i32[]})
        n72 = control-ref of="LIN_Data_display"() -> (w143:refnum<vi>)
        n73 = And Array Elements(Boolean array=w146) -> (logical AND=→"result 2":bool)
        n74 = call "TSLIN_Schedule_Table_Display.vi"("LIN Scheduling Table Array"=w142, "LIN_Data Ref"=w143) -> ()  [unwired: 9 in, 1 out]
      }
      frame "Clear CH" {
        n75 = Unbundle By Name(w158) -> ("Data.LIN_Data.DLL_PATH"=w163:path)
        n76 = Unbundle By Name(w158) -> ("Data.LIN_Data.LIN Scheduling Table Array"=w157:T9[])
        n77 = local read "LIN scheduling table"() -> (w159:T9)
        n78 = Unbundle By Name(w159) -> ("LIN_Transmit.Channel"=w155:i32)
        n79 = for {
          tunnel: w157 -> [w166] mode=indexing
          tunnel: w155 -> [w167]
          tunnel: [w166] -> w154 mode=indexing if=w164
          n80 = Unbundle By Name(w166) -> ("LIN_Transmit.Channel"=w168:i32)
          n81 = Equal?(x=w168, y=w167) -> (x = y?=w165:bool)
          n82 = Not(x=w165) -> (.not. x?=w164:bool)
        }
        n83 = call "tslin_clear_schedule_tables.vi"("ALdxChn"=w155, "路径输入"=w163) -> ("return"=w161:i32)  [unwired: 7 in, 2 out]
        n84 = control-ref of="LIN_Data_display"() -> (w162:refnum<vi>)
        n85 = Equal To 0?(x=w161) -> (x = 0?=→"result 3":bool)
        n86 = Bundle By Name(cluster=w158, "Data.LIN_Data.LIN Scheduling Table Array"=w154) -> (w156:cluster{"Data":T1, "Channel array":i32[]})
        n87 = call "TSLIN_Schedule_Table_Display.vi"("LIN Scheduling Table Array"=w154, "LIN_Data Ref"=w162) -> ()  [unwired: 9 in, 1 out]
      }
      frame "Quit" {
        n88 = Flush Queue(queue=w172, error in (no error)=w170) -> (queue out=w173:refnum<queue>, error out=w171:errorcluster)  [unwired: 1 out]
      }
    }
    n89 = Unbundle By Name(w53) -> ("message"=w52:string)
    n90 = case shown="\"default\", 默认" w52 {
      tunnel: w59 -> [w70 w72]
      tunnel: w58 -> [w69 w71]
      tunnel: w53 -> [w68 _]
      tunnel: [w67 w72] -> w56
      tunnel: [w66 w71] -> w55
      frame "default", Default {
        n91 = Enqueue Element(queue=w70, element=w68, error in (no error)=w69) -> (queue out=w67:refnum<queue>, error out=w66:errorcluster)  [unwired: 1 in, 1 out]
      }
      frame "" {
      }
    }
  }
  n92 = while {
    tunnel: w22 -> [w182]
    tunnel: w15 -> [w180]
    tunnel: "Sender" -> [w176]
    tunnel: w10 -> [w175]
    tunnel: w9 -> [_]
    stop <- w183 stop-if-true
    n93 = event shown="[9] \"Signals\": 值改变" {
      selector: w175 -> [_ _ _ _ _ _ _ _ _ _]
      dyn-events: _ -> [_ _ _ _ _ _ _ _ _ _]
      timeout: _ -> [_ _ _ _ _ _ _ _ _ _]
      tunnel: [_ w194 w201 TRUE ("放弃？") _ _ _ _ _ _] -> w183
      tunnel: w182 -> [w193 w197 w200 w204 w218 w222 w226 w232 w238 w244]
      tunnel: [w193 w197 w198 w202 w218 w222 w226 w232 w238 w244] -> w181
      tunnel: [T13 {"Sender"="", "receiver"="", "message"="", "data"=variant} ("Communication message") _ _ _ w215 w219 w223 w229 w234 w240] -> w178
      tunnel: [w192 _ _ _ _ _ _ _ _ _] -> w179
      tunnel: w180 -> [w192 _ _ _ _ _ _ _ _ _]
      tunnel: w176 -> [_ _ _ _ _ _ _ _ _ _]
      event Timeout {
        n94 = event-data() -> ()  [unwired: 1 in, 3 out]
      }
      event User Event {
        n95 = event-data() -> ("Exit"=w196:string)  [unwired: 1 in]
        n96 = Equal?(x=w196, y="Exit") -> (x = y?=w194:bool)
      }
      event Panel Close? {
        w201 = TRUE ("放弃？")
        n97 = event-data() -> ()  [unwired: 1 in, 4 out]
        n98 = Enqueue Element(queue=w200, element=T13 {"Sender"="", "receiver"="", "message"="Quit", "data"=variant} ("Communication message")) -> (queue out=w198:refnum<queue>)  [unwired: 2 in, 2 out]
        n99 = event-data("Discard?"=w201) -> ()  [unwired: 1 in, 1 out]
      }
      event "Confirm": Value Change {
        n100 = event-data() -> ()  [unwired: 1 in, 6 out]
        n101 = Enqueue Element(queue=w204, element=T13 {"Sender"="", "receiver"="", "message"="Quit", "data"=variant} ("Communication message")) -> (queue out=w202:refnum<queue>)  [unwired: 2 in, 2 out]
      }
      event Value Change {
        n102 = event-data() -> ()  [unwired: 1 in, 6 out]
        n103 = local read "LIN scheduling table"() -> (w212:T9)
        n104 = Unbundle By Name(w212) -> ("LIN_Transmit.Channel"=w211:i32, "LIN_Transmit.Rx/TX"=w208:enum16{"Rx", "Tx"}, "LIN_Transmit.Set_node_funtiontype"=w206:i32, "LIN_Transmit.DLC"=w209:u32, "LIN_Transmit.ID"=w210:u32, "LIN_Transmit.FDatas"=w207:T23)
        n105 = Bundle By Name(cluster=T1 {"Communication message"={"Sender"="", "receiver"="", "message"="", "data"=variant}, "LIN_Data"={"DLL_PATH"=path "", "Channels used"=0, "Funtiontype"=0, "Rx/TX"=enum."Rx", "Read message type"=enum."Only read received messages", "async&sync"=enum."async", "sync_sendTimeout"=0, "LIN_SendHead"={"ALINIdxchn"=0, "ALINId"=0, "ALINDLC"=0}, "LIN_Set"={"Hardware Type"=0, "Hardware Subtype"=enum."TS_UNKNOWN_DEVICE", "AHwChannel"=0, "AAppChannel"=0, "ABaudrateKbps"=0.0, "AProtocol"=0, "AldHW"=0}, "LIN_DATA"={"Data0"=0, "Data1"=0, "Data2"=0, "Data3"=0, "Data4"=0, "Data5"=0, "Data6"=0, "Data7"=0}, "LIN_Set_Array"=[], "LDF"={"LDF Path"=path "", "LDF loading channel"=0}, "Blf_Log"={"Blf_Log_PATH"=path ""}, "LIN Scheduling Table Array"=[], "REC_Channel"=0}, "LIN Data array"=[], "error in"={"status"=FALSE, "code"=0, "source"=""}, "REC_Channel"=0, "AsynCall?"=FALSE, "DataBase_array"=refnum} ("Data"), "LIN_Data.LIN_SendHead.ALINIdxchn"=w211, "LIN_Data.LIN_SendHead.ALINId"=w210, "LIN_Data.LIN_SendHead.ALINDLC"=w209, "LIN_Data.Rx/TX"=w208, "LIN_Data.LIN_DATA"=w207, "LIN_Data.Funtiontype"=w206) -> (w213:T1)
        n106 = Bundle By Name(cluster=T13 {"Sender"="", "receiver"="", "message"="", "data"=variant} ("Communication message"), "message"="Config update", "data"=w213) -> (w215:T13)
      }
      event "Clear all": Value Change {
        n107 = event-data() -> ()  [unwired: 1 in, 6 out]
        n108 = Bundle By Name(cluster=T13 {"Sender"="", "receiver"="", "message"="", "data"=variant} ("Communication message"), "message"="Clear") -> (w219:T13)
      }
      event "Clear CH": Value Change {
        # "Clear the current designated channel"
        n109 = event-data() -> ()  [unwired: 1 in, 6 out]
        n110 = Bundle By Name(cluster=T13 {"Sender"="", "receiver"="", "message"="", "data"=variant} ("Communication message"), "message"="Clear CH") -> (w223:T13)
      }
      event "Add": Value Change {
        n111 = event-data() -> ()  [unwired: 1 in, 6 out]
        n112 = To Variant(anything="LIN scheduling table") -> (Variant=w227:variant)
        n113 = Bundle By Name(cluster=T13 {"Sender"="", "receiver"="", "message"="", "data"=variant} ("Communication message"), "message"="Add", "data"=w227) -> (w229:T13)
      }
      event "Messages": Value Change {
        n114 = event-data() -> ("NewVal"=w233:string)  [unwired: 1 in, 5 out]
        n115 = To Variant(anything=w233) -> (Variant=w235:variant)
        n116 = Bundle By Name(cluster=T13 {"Sender"="", "receiver"="", "message"="", "data"=variant} ("Communication message"), "message"="Messages" ("Sender"), "data"=w235) -> (w234:T13)
      }
      event "Signals": Value Change {
        n117 = event-data() -> ("NewVal"=w239:string[][])  [unwired: 1 in, 5 out]
        n118 = To Variant(anything=w239) -> (Variant=w241:variant)
        n119 = Bundle By Name(cluster=T13 {"Sender"="", "receiver"="", "message"="", "data"=variant} ("Communication message"), "message"="Signals" ("Sender"), "data"=w241) -> (w240:T13)
      }
    }
    n120 = Unbundle By Name(w178) -> ("message"=w177:string)
    n121 = case shown="\"default\", 默认" w177 {
      tunnel: w181 -> [w188 w190]
      tunnel: w179 -> [w187 w189]
      tunnel: w178 -> [w186 _]
      tunnel: [w185 w190] -> _
      tunnel: [w184 w189] -> _
      frame "default", Default {
        n122 = Enqueue Element(queue=w188, element=w186, error in (no error)=w187) -> (queue out=w185:refnum<queue>, error out=w184:errorcluster)  [unwired: 1 in, 1 out]
      }
      frame "" {
      }
    }
  }
  n123 = Release Queue(queue=w21, error in (no error)=w20) -> (error out=w19:errorcluster)  [unwired: 1 in, 2 out]
  n124 = Unbundle By Name(w7) -> ("Data.LIN_Data.LIN Scheduling Table Array"=w6:T9[])
  n125 = property class="App"(error in=w19) -> (error out=w18:errorcluster, "App.Kind"=w17:T24)  [unwired: 1 in, 1 out]
  n126 = case shown="\"Run Time System\"" w17 {
    tunnel: w18 -> [_ _ w245 _ _ _ _]
    frame "invalid app kind", Default {
    }
    frame "Development System" {
    }
    frame "Run Time System" {
      n127 = invoke class="VI" method="FP.Close"(error in=w245) -> ()  [unwired: 2 in, 3 out]
    }
    frame "Student Edition" {
    }
    frame "Embedded LabVIEW" {
    }
    frame "Evaluation" {
    }
    frame "Custom" {
    }
  }
  n128 = Bundle By Name(cluster=w4, "LIN_Data.LIN Scheduling Table Array"=w6, "Communication message"=w1) -> (→"Data out":T1)
  "错误输出" <- w9
